vi "Launch Depth Actor.vi"(11 "RDS Root Actor in":refnum<class "RDS Root Actor.lvclass">) -> (3 "RDS Root Actor out":refnum<class "RDS Root Actor.lvclass">)   [LabVIEW 2015, in "RDS Root Actor.lvlib" / "RDS Root Actor.lvclass"]
uses:
  RDS Root Actor.lvclass
  Libraries/RDS Framework/RDS Message ID.ctl
  Depth Instrument/Depth Instrument/Depth Instrument.lvclass
  Libraries/RDS Instruments/RDS Instrument Enums.ctl
  RDS Parent Actor/RDS Parent Actor/RDS Parent Actor.lvclass/RDS Parent Actor.ctl
  RDS Serial Instrument Actor/RDS Serial Instrument Actor.lvclass/RDS Serial Instrument Actor.ctl
  RDS Parent Actor/RDS Parent Actor/RDS Parent Actor.lvclass
  RDS Serial Instrument Actor/RDS Serial Instrument Actor.lvclass
  Libraries/RDS Child Messages/RDS Child Messages.lvlib
  Libraries/Configuration Library/RDS Configuration Library.lvlib
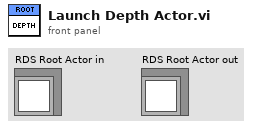
[diagram p1: front panel]
types:
  T1 = typedef "RDS Configuration Library.lvlib/RDS Instrument Enums.ctl" = enum16{"AIP", "GPS", "Compass", "PORT Motor", "STBD Motor", "LSR", "Depth Transducer", "BTB"}
  T2 = typedef "RDS Child Messages.lvlib/RDS Message ID.ctl" = enum16{"RDS Hello World", "String Message", "AIP_Status", "AIP_Command", "GPS_Data", "MCB_Command", "MCB_Status", "Compass_Data", "Depth_Data", "Battery_Data", "Contoller_State", "Set_Mag_Dev", "BTB_Shutdown", "State_Sample_Request", "State_Sample", "PID_Gains_Set", "Helm_Limiter_Set", "Helm_Heading_Command", "Helm_Steering_Command", "Helm_Status", "Controller_Message", "AIP_Set_Min_Depth", "Mission_Controller_State", "Mission_Upload", "Mission_Set_Op_and_Run", "Mission_Settings_Set"}
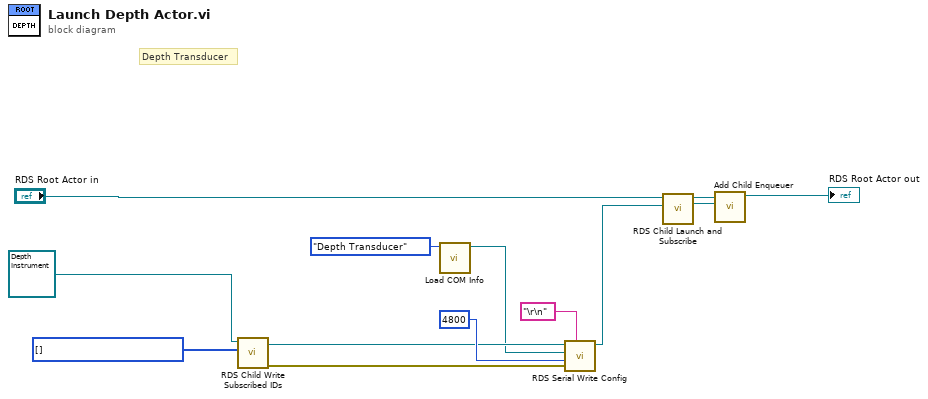
[diagram p0: block diagram]
diagram:
  w6 = T2[] [] items=["RDS Hello World", "String Message", "AIP_Status", "AIP_Command", "GPS_Data", "MCB_Command", "MCB_Status", "Compass_Data", "Depth_Data", "Battery_Data", "Contoller_State", "Set_Mag_Dev", "BTB_Shutdown", "State_Sample_Request", "State_Sample", "PID_Gains_Set", "Helm_Limiter_Set", "Helm_Heading_Command", "Helm_Steering_Command", "Helm_Status", "Controller_Message", "AIP_Set_Min_Depth", "Mission_Controller_State", "Mission_Upload", "Mission_Set_Op_and_Run", "Mission_Settings_Set"] ("Subscribed IDs")
  # "Depth Transducer"
  n1 = call "RDS Child Write Subscribed IDs.vi"("Subscribed IDs"=w6, "RDS Parent Actor in"=refnum<class "Depth Instrument.lvclass"> refnum ("Depth Instrument.lvlib:Depth Instrument.lvclass")) -> ("error out"=w5:errorcluster, "RDS Parent Actor out"=w4:refnum<class "Depth Instrument.lvclass">)  [unwired: 8 in]
  n2 = call "Load COM Info.vi"("Serial Instrument"=RDS_Instrument_Enums."Depth Transducer") -> ("COM Port"=w1:refnum<visa-resource-name>)  [unwired: 10 in]
  n3 = call "RDS Serial Write Config.vi"("Termination Char(s)"="\r\n", "error in (no error)"=w5, "baud rate"=u32 4800, "VISA resource name"=w1, "RDS Serial Instrument Actor in"=w4) -> ("RDS Serial Instrument Actor out"=w9:refnum<class "Depth Instrument.lvclass">)  [unwired: 5 in, 1 out]
  n4 = call "RDS Child Launch and Subscribe.vi"("RDS Child in"=w9, "Caller Actor in"="RDS Root Actor in") -> ("Nested Actor's Enqueuer"=w12:refnum<class "Message Enqueuer.lvclass">, "Caller Actor Out"=w11:refnum<class "RDS Root Actor.lvclass">)  [unwired: 7 in, 1 out]
  n5 = call "Add Child Enqueuer.vi"("Nested Actor's Enqueuer"=w12, "RDS Root Actor in"=w11) -> ("RDS Root Actor out"=→"RDS Root Actor out":refnum<class "RDS Root Actor.lvclass">)  [unwired: 8 in, 1 out]
